vi "Test Set Cell Value.vi"(11 "Test Case In":refnum<class "Test Open Xml.lvclass">) -> (0 "error out":errorcluster, 3 "Test Case Out":refnum<class "Test Open Xml.lvclass">)   [LabVIEW 2021, in "Test Open Xml.lvclass"]
uses:
  Test Open Xml.lvclass
  Test Open Xml.lvclass/Test Open Xml.ctl
  Source/Open Xml.lvlib
  <vilib>/Astemes/LUnit/Test Case.lvclass
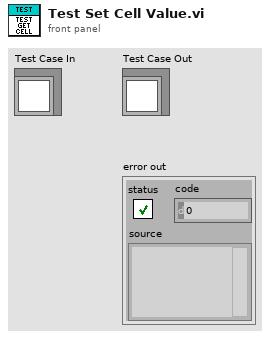
[diagram p1: front panel]
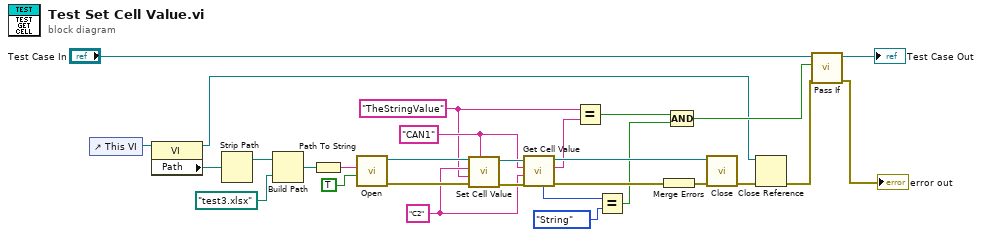
[diagram p0: block diagram]
diagram:
  w9 = "C2" ("Cell Address")
  w10 = "CAN1" ("Sheet Name")
  w8 = "TheStringValue"
  n1 = control-ref of="This VI"() -> (w26:refnum<vi>)
  n2 = property class="VI"(reference=w26) -> (reference out=w1:refnum<vi>, "Path"=w25:path)  [unwired: 1 in, 1 out]
  n3 = Strip Path(path=w25) -> (stripped path=w24:path)  [unwired: 1 out]
  n4 = Build Path(base path=w24, name or relative path=path "test3.xlsx") -> (appended path=w22:path)
  n5 = Path To String(path=w22) -> (string=w21:string)
  n6 = call "Open.vi"("isEditable"=TRUE, "Path"=w21) -> ("error out"=w12:errorcluster, "SpreadsheetDocument"=w14:refnum<k24>)  [unwired: 8 in]
  n7 = call "Set Cell Value.vi"("Sheet Name"=w10, "error in"=w12, "Value"=w8, "Cell Address"=w9, "SpreadsheetDocument"=w14) -> ("error out"=w11:errorcluster, "SpreadsheetDocument out"=w13:refnum<k24>)  [unwired: 5 in]
  n8 = call "Get Cell Value.vi"("error in"=w11, "Cell Address"=w9, "Sheet Name"=w10, "SpreadsheetDocument"=w13) -> ("error out"=w15:errorcluster, "Value String"=w18:string, "SpreadsheetDocument out"=w19:refnum<k24>, "Type"=w5:enum16{"Void", "String", "Numeric", "Boolean"})  [unwired: 2 in, 2 out]
  n9 = Equal?(x=w8, y=w18) -> (x = y?=w7:bool)
  n10 = Equal?(x=w5, y=enum16{"Void", "String", "Numeric", "Boolean"}."String" ("Type")) -> (x = y?=w3:bool)
  n11 = Merge Errors(w15) -> (w17:errorcluster)
  n12 = Compound Arithmetic op=AND(w7, w3) -> (w4:bool)
  n13 = call "Close.vi"("error in"=w17, "SpreadsheetDocument"=w19) -> ("error out"=w16:errorcluster)  [unwired: 9 in]
  n14 = Close Reference(reference=w1, error in (no error)=w16) -> (error out=w2:errorcluster)
  n15 = call <vilib>:"Pass If.vi"("error in (no error)"=w2, "Pass?"=w4, "LUnit Test Case In"="Test Case In") -> ("error out"=→"error out":errorcluster, "LUnit Test Case Out"=→"Test Case Out":refnum<class "Test Open Xml.lvclass">)  [unwired: 7 in]
